vi "Send Write Setup.vi"(8 "error in (no error)":errorcluster, 11 "RxTx in":refnum<class "RxTx.lvclass">) -> (0 "error out":errorcluster, 3 "RxTx out":refnum<class "RxTx.lvclass">)   [LabVIEW 2018, in "RxTx.lvclass"]
uses:
  RxTx.lvclass
  Interface/Interface.lvclass
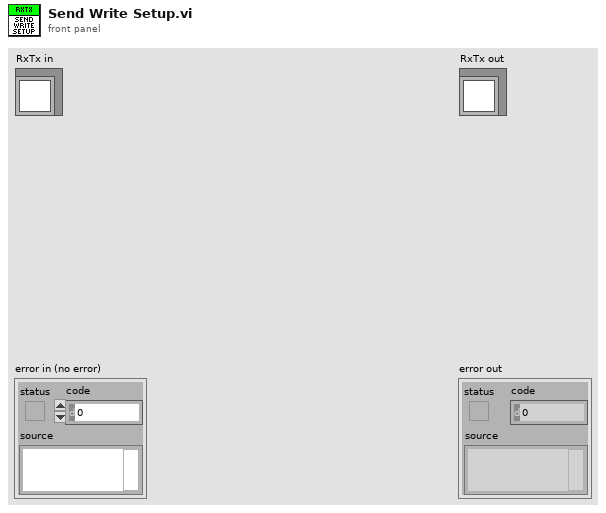
[diagram p1: front panel]
types:
  T1 = typedef "Shutter_mode typedef.ctl" = enum16{"Auto", "Open", "Close", "N/A (3)", "Open FVB Series", "Open Any Series"}
  T2 = typedef "ReadMode_mode typedef.ctl" = enum16{"Full Vertical Binning", "Multi-Track", "Random-Track", "Single-Track", "Image"}
  T3 = typedef "AcquisitionMode_mode typedef.ctl" = enum16{"Reserved (0)", "Single Scan", "Accumulate", "Kinetics", "Fast Kinetics", "Run Till Abort", "Reserved (6)", "Reserved (7)", "Reserved (8)", "Time Delayed Integration"}
  T4 = cluster{"EXPTIME":sgl, "PREAMP":enum16{"Gain 1", "Gain 2"}, "READOUT_RATE":enum16{"1 MHz", "10 MHz", "20 MHz", "30 MHz"}, "EM_MODE":enum16{"Electron Multiplying", "Conventional"}, "EM_GAIN":u16, "VBIN":u16, "INITIAL_LINE":u16, "INITIAL_COLUMN":u16, "FINAL_LINE":u16, "FINAL_COLUMN":u16, "#FRAMES":u32, "#CUBES":u32, "TRIGGER_MODE":u16, "HBIN":u16, "SHUTTER_TTL":enum16{""}, "SHUTTER_MODE":T1, "SHUTTER_OPENING_TIME":u16, "SHUTTER_CLOSING_TIME":u16, "VERTICAL_SHIFT_SPEED":u16, "READ_MODE":T2, "FRAME_TRANSFER":bool, "VERTICAL_CLOCK_VOLTAGE":enum16{"0", "+1", "+2", "+3", "+4"}, "ACQUISITION_MODE":T3, "AD_CHANNEL":u16}
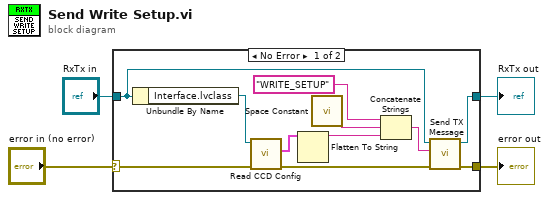
[diagram p0: block diagram]
diagram:
  n1 = case shown="No Error" "error in (no error)" {
    selector: "error in (no error)" -> [w14 w17]
    tunnel: [w8 w17] -> w2
    tunnel: [w9 w16] -> w1
    tunnel: "RxTx in" -> [w10 w16]
    frame No Error {
      n2 = Unbundle By Name(w10) -> ("Interface.lvclass"=w15:refnum<class "Interface.lvclass">)
      n3 = call "Read CCD Config.vi"("error in (no error)"=w14, "Interface in"=w15) -> ("error out"=w12:errorcluster, "CCD Config"=w6:T4)  [unwired: 7 in, 1 out]
      n4 = Flatten To String(anything=w6) -> (data string=w13:string)  [unwired: 3 in, 2 out]
      n5 = call <vilib>:"Space Constant.vi"() -> ("String"=w7:string)
      n6 = Concatenate Strings("WRITE_SETUP", w7, w13) -> (w11:string)
      n7 = call "Send TX Message.vi"("error in (no error)"=w12, "element"=w11, "RxTx in"=w10) -> ("error out"=w8:errorcluster, "RxTx out"=w9:refnum<class "RxTx.lvclass">)  [unwired: 7 in]
    }
    frame Error {
    }
  }
  "error out" <- w2
  "RxTx out" <- w1
